vi "LimeLight.vi"() -> ()   [LabVIEW 2018]
panel:
  out "Correction":dbl
  in  "Max Output":cluster{"output high":dbl, "output low":dbl}={"output high"=100.0, "output low"=-100.0} {"output low" format="%.2f"; "output high" format="%.2f"}
  in  "PID gains":T1={"proportional gain (Kc)"=1.0, "integral time (Ti, min)"=0.01, "derivative time (Td, min)"=0.0} {"derivative time (Td, min)" format="%.3f"; "integral time (Ti, min)" format="%.3f"; "proportional gain (Kc)" format="%.3f"}
  out "WriteCamera":T2
  out "ReadCamera":T3
  out "CameraInfo":cluster{"Processing?":bool, "IP & Port":string}
  out "CameraData":T4
  # "From CrossHair"
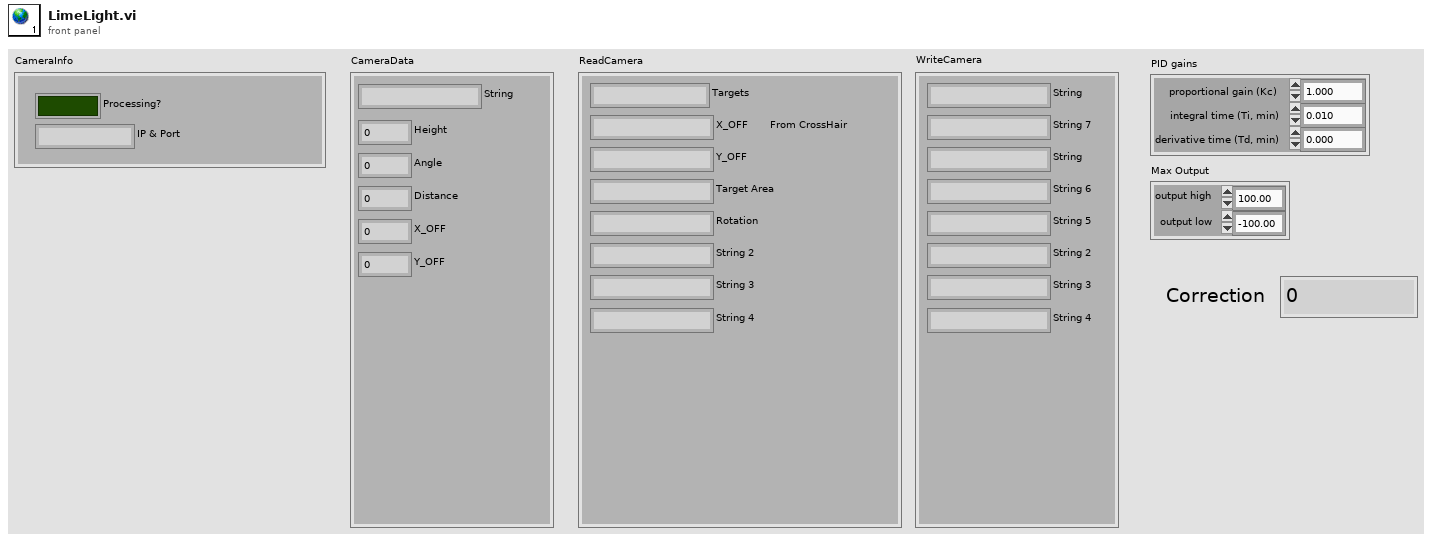
[diagram p1: front panel]
types:
  T1 = cluster{"proportional gain (Kc)":dbl, "integral time (Ti, min)":dbl, "derivative time (Td, min)":dbl}
  T2 = cluster{"String":string, "String":string, "String 2":string, "String 3":string, "String 4":string, "String 5":string, "String 6":string, "String 7":string}
  T3 = cluster{"Targets ":string, "Y_OFF":string, "String 2":string, "String 3":string, "String 4":string, "Rotation":string, "Target Area":string, "X_OFF":string}
  T4 = cluster{"String":string, "Height":dbl, "Angle":dbl, "Distance":dbl, "X_OFF":dbl, "Y_OFF":dbl}
diagram:
